vi "Build NT Data Update for Cluster.vi"(10 "Field Value":T1, 11 "Field ID":T4) -> (3 "Data Buffer":string)   [LabVIEW 2017]
uses:
  <vilib>/Rock Robotics/Network Tables/Field ID.ctl
  <vilib>/Rock Robotics/Network Tables/Field Data.ctl
  <vilib>/Rock Robotics/Network Tables/Field Type.ctl
  <vilib>/Rock Robotics/Network Tables/Sequence.ctl
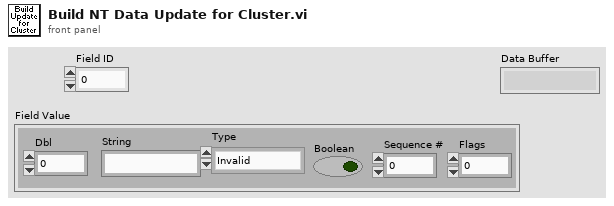
[diagram p1: front panel]
types:
  T1 = typedef "Field Data.ctl" = cluster{"Dbl":dbl, "String":string, "Type":T2, "Boolean":bool, "Sequence #":T3, "Flags":u8}
  T2 = typedef "Field Type.ctl" = enum8{"Invalid", "Bool", "Numeric", "String", "Raw", "Boolean Array", "Numeric Array", "String Array", "RPC"}
  T3 = typedef "Sequence.ctl" = u16
  T4 = typedef "Field ID.ctl" = i32
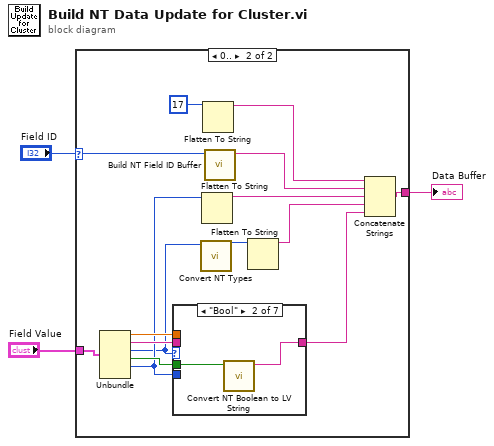
[diagram p0: block diagram]
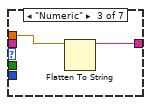
[diagram p4: hidden frame]
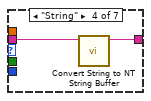
[diagram p5: hidden frame]
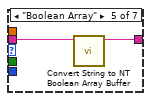
[diagram p6: hidden frame]
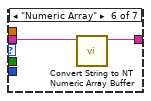
[diagram p7: hidden frame]
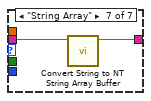
[diagram p8: hidden frame]
diagram:
  n1 = case shown="0.." "Field ID" {
    selector: "Field ID" -> [_ w8]
    tunnel: "Field Value" -> [_ w16]
    tunnel: [_ w9] -> w2
    frame Default {
    }
    frame 0.. {
      n2 = Unbundle(w16) -> ("Dbl"=w18:dbl, "String"=w17:string, "Type"=w7:T2, "Boolean"=w15:bool, "Sequence #"=w10:T3)  [unwired: 1 out]
      n3 = case shown="\"Bool\"" w7 {
        tunnel: w10 -> [_ _ _ _ _ _ _]
        tunnel: w17 -> [_ _ _ w24 w25 w27 w29]
        tunnel: [_ w19 w21 w23 w26 w28 w30] -> w5
        tunnel: w18 -> [_ _ w22 _ _ _ _]
        tunnel: w15 -> [_ w20 _ _ _ _ _]
        frame Default {
        }
        frame "Bool" {
          n4 = call <vilib>:"Convert NT Boolean to LV String.vi"("Boolean"=w20) -> ("string"=w19:string)  [unwired: 10 in]
        }
        frame "Numeric" {
          n5 = Flatten To String(anything=w22) -> (data string=w21:string)  [unwired: 3 in, 2 out]
        }
        frame "String" {
          n6 = call <vilib>:"Convert String to NT String Buffer.vi"("LV Buffer"=w24) -> ("NT Buffer"=w23:string)  [unwired: 10 in]
        }
        frame "Boolean Array" {
          n7 = call <vilib>:"Convert String to NT Boolean Array Buffer.vi"("LV Buffer"=w25) -> ("NT Buffer"=w26:string)  [unwired: 10 in]
        }
        frame "Numeric Array" {
          n8 = call <vilib>:"Convert String to NT Numeric Array Buffer.vi"("LV Buffer"=w27) -> ("NT Buffer"=w28:string)  [unwired: 10 in]
        }
        frame "String Array" {
          n9 = call <vilib>:"Convert String to NT String Array Buffer.vi"("LV Buffer"=w29) -> ("NT Buffer"=w30:string)  [unwired: 10 in]
        }
      }
      n10 = call <vilib>:"Convert NT Types.vi"("Type in"=w7) -> ("Type out"=w6:u8)  [unwired: 10 in]
      n11 = Flatten To String(anything=w10) -> (data string=w14:string)  [unwired: 3 in, 2 out]
      n12 = Flatten To String(anything=u8 17 ("bytes to read")) -> (data string=w13:string)  [unwired: 3 in, 2 out]
      n13 = call <vilib>:"Build NT Field ID Buffer.vi"("Field ID"=w8) -> ("Data Buffer"=w11:string)  [unwired: 10 in]
      n14 = Flatten To String(anything=w6) -> (data string=w4:string)  [unwired: 3 in, 2 out]
      n15 = Concatenate Strings(w13, w11, w14, w4, w5) -> (w9:string)
    }
  }
  "Data Buffer" <- w2
